vi "Timing Report.vi"   [LabVIEW 2014]
uses:
  <vilib>/Utility/error.llb/DialogType.ctl
  <vilib>/gmath/statdist.llb/st_Percentiles (scalar).vi
  <vilib>/gmath/NI_Gmath.lvlib
  <vilib>/Wiresmith Technology/LabVIEW CLI/CLI Class/CLI.lvclass
types:
  T1 = typedef "DialogType.ctl" = u16
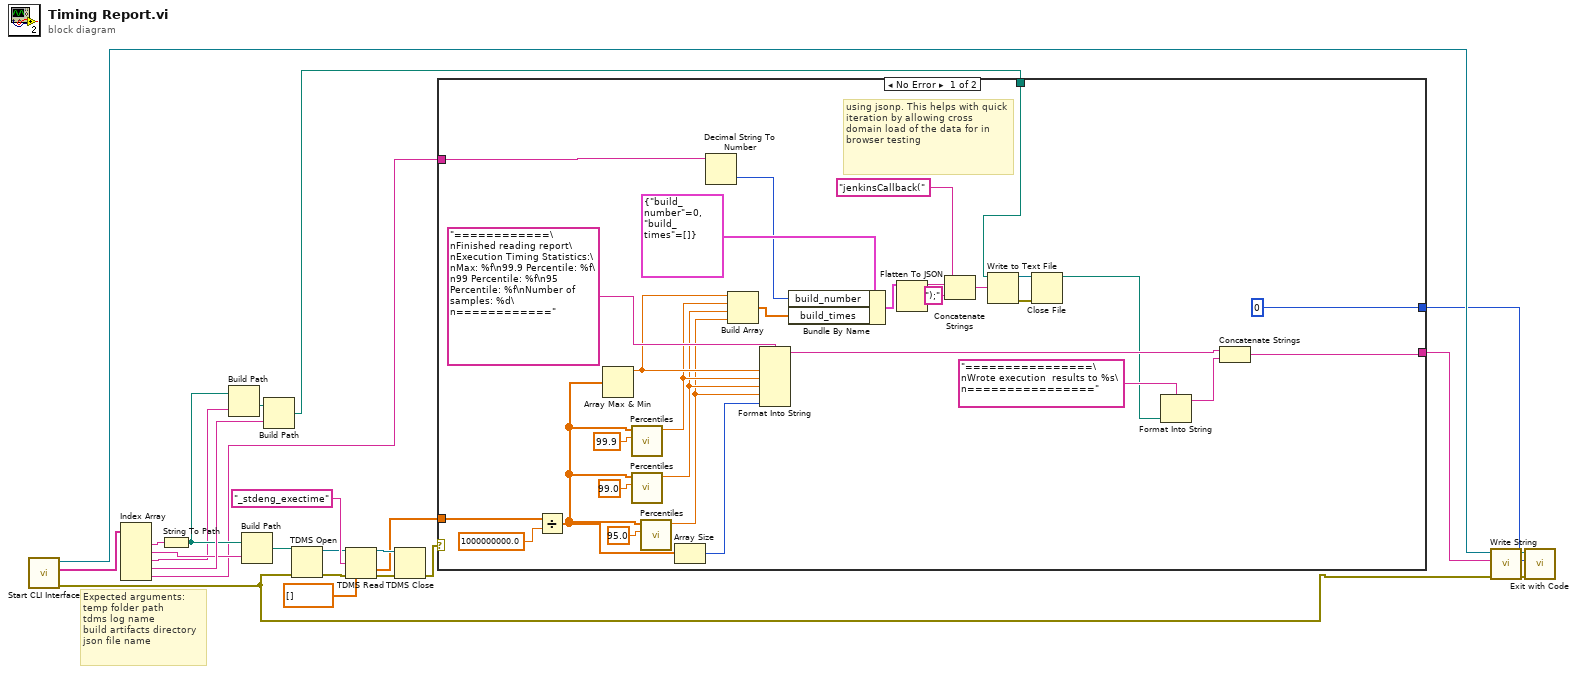
[diagram p0: block diagram]
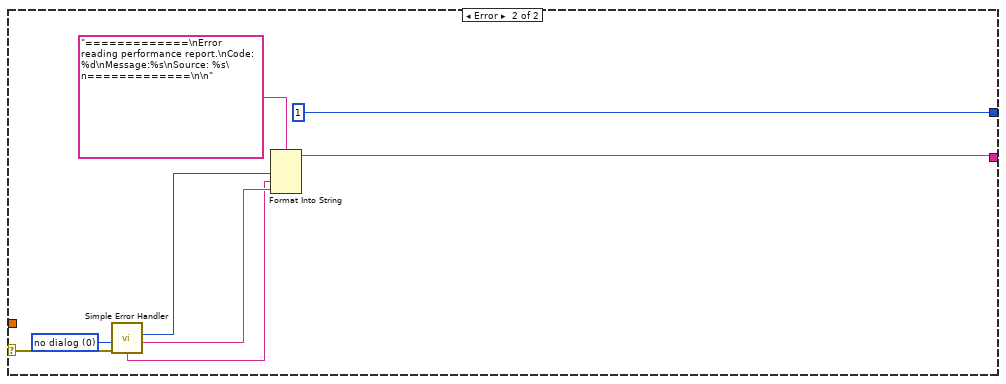
[diagram p2: hidden frame]
diagram:
  # "Expected arguments:\ntemp folder path\ntdms log name\nbuild artifacts directory\njson file name"
  n1 = call <vilib>:"Start CLI Interface.vi"() -> ("error out"=w9:errorcluster, "Custom Parameters"=w17:string[], "CLI out"=w12:refnum<class "CLI.lvclass">)  [unwired: 9 in]
  n2 = Index Array(array=w17) -> (element #1=w16:string, element #2=w3:string, element #3=w2:string, element #4=w7:string, element #5=w1:string)  [unwired: 5 in]
  n3 = String To Path(string=w16) -> (path=w4:path)
  n4 = Build Path(base path=w4, name or relative path=w2) -> (appended path=w5:path)
  n5 = Build Path(base path=w4, name or relative path=w3) -> (appended path=w8:path)
  n6 = Build Path(base path=w5, name or relative path=w7) -> (appended path=w6:path)
  n7 = TDMS Open(8:w9, 11:w8) -> (0:w19:errorcluster, 3:w18:refnum<k34>)  [unwired: 5 in]
  n8 = TDMS Read(0:w18, 7:"_stdeng_exectime" ("channel name(s) in"), 11:w19, 12:dbl[] []) -> (4:w24:refnum<k34>, 10:w22:dbl[], 15:w23:errorcluster)  [unwired: 4 in, 3 out]
  n9 = TDMS Close(8:w23, 11:w24) -> (0:w10:errorcluster)  [unwired: 1 out]
  n10 = case shown="No Error" w10 {
    selector: w10 -> [_ w59]
    tunnel: w22 -> [w54 _]
    tunnel: [w42 w55] -> w13
    tunnel: [0 ("Exit Code (0)") 1 ("Exit Code (0)")] -> w11
    tunnel: w6 -> [w39 _]
    tunnel: w1 -> [w31 _]
    frame No Error {
      # "using jsonp. This helps with quick iteration by allowing cross domain load of the data for in browser testing"
      n11 = Divide(x=w54, y=1000000000.0) -> (x/y=w26:dbl[])
      n12 = Array Max & Min(array=w26) -> (max value=w47:dbl)  [unwired: 3 out]
      n13 = call-poly <vilib>:"Percentiles.vi"("p"=99.9, "x array"=w26) -> ("percentile"=w46:dbl)  [unwired: 8 in, 1 out]
      n14 = call-poly <vilib>:"Percentiles.vi"("p"=99.0, "x array"=w26) -> ("percentile"=w45:dbl)  [unwired: 8 in, 1 out]
      n15 = call-poly <vilib>:"Percentiles.vi"("p"=95.0, "x array"=w26) -> ("percentile"=w44:dbl)  [unwired: 8 in, 1 out]
      n16 = Array Size(array=w26) -> (size(s)=w25:i32)
      n17 = Decimal String To Number(string=w31) -> (number=w29:i32)  [unwired: 2 in, 1 out]
      n18 = Build Array(w47, w46, w45, w44) -> (w28:dbl[])
      n19 = Format Into String(format string="============\nFinished reading report\nExecution Timing Statistics:\nMax: %f\n99.9 Percentile: %f\n99 Percentile: %f\n95 Percentile: %f\nNumber of samples: %d\n============", w47, w46, w45, w44, w25) -> (resulting string=w41:string)  [unwired: 2 in, 1 out]
      n20 = Bundle By Name(cluster=cluster{"build_number":i32, "build_times":dbl[]} {"build_number"=0, "build_times"=[]}, "build_number"=w29, "build_times"=w28) -> (w27:cluster{"build_number":i32, "build_times":dbl[]})
      n21 = Flatten To JSON(anything=w27) -> (JSON string=w34:string)  [unwired: 2 in, 1 out]
      n22 = Concatenate Strings("jenkinsCallback(" ("string"), w34, ");" ("string")) -> (w35:string)
      n23 = Write to Text File(file (use dialog)=w39, text=w35) -> (refnum out=w37:refnum<file>, error out=w38:errorcluster)  [unwired: 2 in, 1 out]
      n24 = Close File(refnum=w37, error in=w38) -> (path=w36:path)  [unwired: 1 out]
      n25 = Format Into String(format string="================\nWrote execution  results to %s\n================", w36) -> (resulting string=w40:string)  [unwired: 2 in, 1 out]
      n26 = Concatenate Strings(w41, w40) -> (w42:string)
    }
    frame Error {
      w60 = T1 0 items=["no dialog", "OK message", "continue or stop message", "OK message + warnings", "continue/stop + warnings"] ("type of dialog (OK msg:1)")
      n27 = call <vilib>:"Simple Error Handler.vi"("type of dialog (OK msg:1)"=w60, "error in (no error)"=w59) -> ("code out"=w58:i32, "source out"=w57:string, "message"=w56:string)  [unwired: 3 in, 2 out]
      n28 = Format Into String(format string="=============\nError reading performance report.\nCode: %d\nMessage:%s\nSource: %s\n=============\n\n", w58, w56, w57) -> (resulting string=w55:string)  [unwired: 2 in, 1 out]
    }
  }
  n29 = call <vilib>:"Write String.vi"("error in (no error)"=w9, "Text to Write"=w13, "CLI in"=w12) -> ("error out"=w15:errorcluster, "CLI out"=w14:refnum<class "CLI.lvclass">)  [unwired: 7 in]
  n30 = call <vilib>:"Exit with Code.vi"("error in (no error)"=w15, "Exit Code (0)"=w11, "CLI in"=w14) -> ()  [unwired: 8 in, 1 out]
